vi "FTW-Subscription-AddAddresses.vi"(0 "FTW-Subscription In":refnum<class "FTW-Subscription.lvclass">, 5 "Addresses":string, 11 "error in (no error)":errorcluster) -> (4 "FTW-Subscription Out":refnum<class "FTW-Subscription.lvclass">, 15 "error out":errorcluster)   [LabVIEW 2013, in "FTW-Subscription.lvclass"]
uses:
  FTW-Subscription.lvclass
  Ether/FTW-Ether-EndpointType.ctl
  Ether/FTW-Ether.lvclass
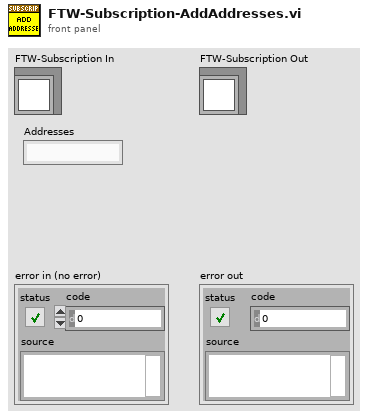
[diagram p1: front panel]
types:
  T1 = typedef "FTW-Ether.lvclass/FTW-Ether-EndpointType.ctl" = enum16{"Server", "Client", "Publisher", "Subscriber"}
  T2 = typedef "FTW-Ether.lvclass/FTW-Ether-MessageTransportScheme.ctl" = enum16{"LabVIEW Queues (lvq://)", "TCP (tcp://)", "LabVIEW Network Streams (lvns://)"}
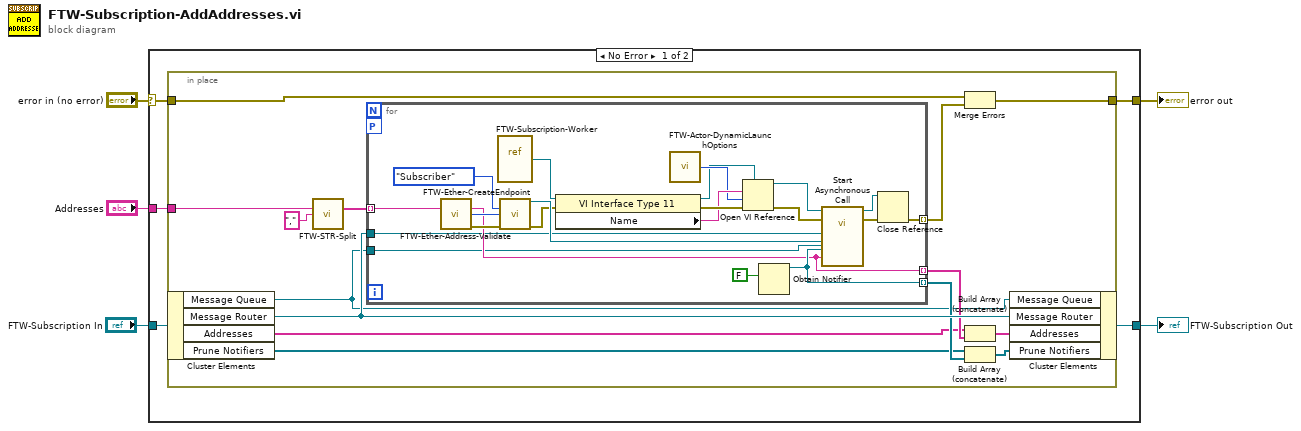
[diagram p0: block diagram]
diagram:
  n1 = case shown="No Error" "error in (no error)" {
    selector: "error in (no error)" -> [w10 w46]
    tunnel: [w9 w46] -> w4
    tunnel: "Addresses" -> [w8 _]
    tunnel: "FTW-Subscription In" -> [w7 w47]
    tunnel: [w6 w47] -> w1
    frame No Error {
      n2 = in-place {
        in-place-border: w10 -> [w24]
        in-place-border: [w23] -> w9
        in-place-border: w8 -> [w20]
        n3 = in-place-cluster #1(w7) -> ("Message Queue"=w11:refnum<queue>, "Message Router"=w18:refnum<user-event>, "Addresses"=w13:string[], "Prune Notifiers"=w12:refnum<notifier>[])
        n4 = call "FTW-STR-Split.vi"("Delimited String"=w20, "Delimiter"=",") -> ("Array of Strings"=w22:string[])  [unwired: 13 in]
        n5 = for {
          tunnel: [w33] -> w19 mode=indexing
          tunnel: w22 -> [w30] mode=indexing
          tunnel: [w29] -> w16 mode=indexing
          tunnel: [w27] -> w17 mode=indexing
          tunnel: w18 -> [w26]
          workers-P: _ -> [_]
          tunnel: w11 -> [w25]
          n6 = call "FTW-Ether-Address-Validate.vi"("Address"=w30) -> ("Sanitized Address"=w27:string, "Message Transport Scheme"=w37:T2, "error out"=w35:errorcluster)  [unwired: 12 in]
          n7 = vi-ref "FTW-Subscription-Worker.vi"() -> (w45:refnum<vi>)
          n8 = call "FTW-Ether-CreateEndpoint.vi"("Endpoint Type"=FTW-Ether-EndpointType."Subscriber", "Message Transport Scheme"=w37, "error in"=w35) -> ("FTW Endpoint"=w31:refnum<class "FTW-Endpoint.lvclass">, "error out"=w28:errorcluster)  [unwired: 11 in]
          n9 = property class="VI Interface Type 11"(reference=w45, error in=w28) -> (reference out=w41:refnum<vi>, error out=w44:errorcluster, "Name"=w43:string)
          n10 = call "FTW-Actor-DynamicLaunchOptions.vi"() -> ("Open VI Ref Options"=w42:i32)
          n11 = Open VI Reference(type specifier VI Refnum (for type only)=w41, vi path=w43, options=w42, error in (no error)=w44) -> (vi reference=w39:refnum<vi>, error out=w34:errorcluster)  [unwired: 2 in]
          n12 = Obtain Notifier(notification data type=FALSE) -> (notifier out=w29:refnum<notifier>)  [unwired: 3 in, 2 out]
          n13 = call-by-ref "Start Asynchronous Call"(reference=w39, error in=w34, "Message Handler"=w26, "Endpoint"=w31, "notifier out"=w29, "Address"=w27, "Queue"=w25) -> (reference out=w38:refnum<vi>, error out=w40:errorcluster)  [unwired: 1 in]
          n14 = Close Reference(reference=w38, error in (no error)=w40) -> (error out=w33:errorcluster)
        }
        n15 = Merge Errors(w24, w19) -> (w23:errorcluster)
        n16 = Build Array (concatenate)(w13, w17) -> (w15:string[])
        n17 = Build Array (concatenate)(w12, w16) -> (w14:refnum<notifier>[])
        n18 = in-place-cluster #1("Message Queue"=w11, "Message Router"=w18, "Addresses"=w15, "Prune Notifiers"=w14) -> (w6:refnum<class "FTW-Subscription.lvclass">)
      }
    }
    frame Error {
    }
  }
  "error out" <- w4
  "FTW-Subscription Out" <- w1
